vi "Construct.vi"(6 "1553 channel handles":T1[](array[typedef]) {"messages"."timestamps" format="%.0x"; "messages"."parameters"."RxBC channel handle" format="%.0x"; "messages"."parameters"."RxRT channel handle" format="%.0x"; "messages"."parameters"."Tx channel handle" format="%.0x"}, 8 "error in":errorcluster, 9 "1553 channels":T5[](array[typedef]), 10 "id":string, 11 "Execution Unit Implementation":refnum<class "Execution Unit.lvclass">) -> (0 "error out":errorcluster, 3 "Execution Unit Implementation out":refnum<class "Execution Unit.lvclass">)   [LabVIEW 2020, in "Ballard MIL-STD-1553 Engine.lvlib" / "Implementation.lvlib" / "Execution Unit.lvclass"]
uses:
  Execution Unit.lvclass
  Shared/1553 Channel.ctl
  Shared/Terminal Name and Address.ctl
  Shared/Address.ctl
  Shared/Message Definition.ctl
  Shared/Message Type.ctl
  Shared/Terminal Endpoint.ctl
  Shared/Parameter Definition.ctl
  Execution Unit.lvclass/Execution Unit.ctl
  <vilib>/NI VeriStand/Custom Device API/Custom Device Item Ref.ctl
  <vilib>/NI VeriStand/Custom Device API/Custom Device API.lvlib
  Parameter Handles.ctl
  Message Handles.ctl
  1553 Channel Handles.ctl
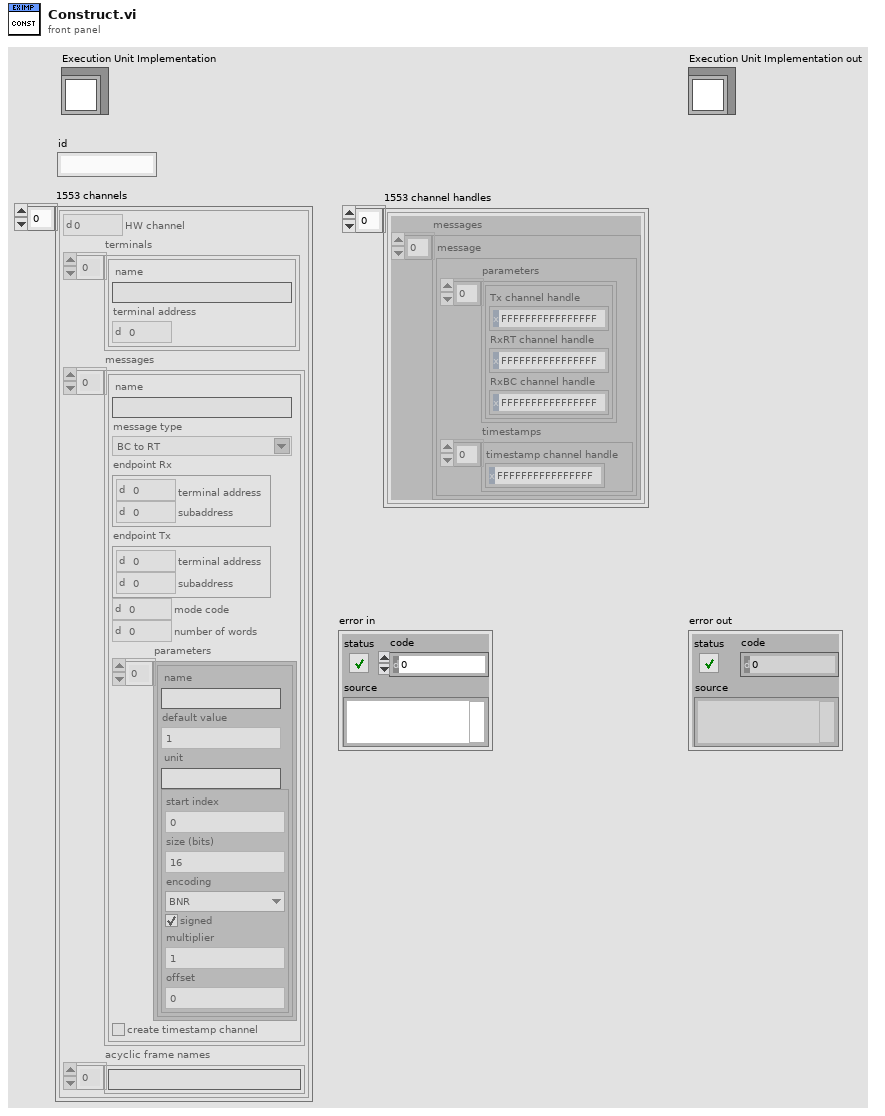
[diagram p1: front panel]
types:
  T1 = typedef "Ballard MIL-STD-1553 Engine.lvlib/Implementation.lvlib/Execution Unit.lvclass/1553 Channel Handles.ctl" = cluster{"messages":T2[]}
  T2 = typedef "Ballard MIL-STD-1553 Engine.lvlib/Implementation.lvlib/Execution Unit.lvclass/Message Handles.ctl" = cluster{"parameters":T3[], "timestamps":T4[]}
  T3 = typedef "Ballard MIL-STD-1553 Engine.lvlib/Implementation.lvlib/Execution Unit.lvclass/Parameter Handles.ctl" = cluster{"Tx channel handle":T4, "RxRT channel handle":T4, "RxBC channel handle":T4}
  T4 = typedef "Custom Device API.lvlib/Custom Device Item Ref.ctl" = u64
  T5 = typedef "1553 Channel.ctl" = cluster{"HW channel":u16, "terminals":T6[], "messages":T8[], "acyclic frame names":string[]}
  T6 = typedef "Terminal Name and Address.ctl" = cluster{"name":string, "terminal address":T7}
  T7 = typedef "Address.ctl" = u16
  T8 = typedef "Message Definition.ctl" = cluster{"name":string, "message type":T9, "endpoint Rx":T10, "endpoint Tx":T10, "mode code":u16, "number of words":u16, "parameters":cluster{"name":string, "default value":dbl, "unit":string, "parameter definition":T11}[], "create timestamp channel":bool}
  T9 = typedef "Message Type.ctl" = string
  T10 = typedef "Terminal Endpoint.ctl" = cluster{"terminal address":T7, "subaddress":T7}
  T11 = typedef "Parameter Definition.ctl" = cluster{"start index":i32, "size (bits)":i32, "encoding":enum16{"BNR", "BCD", "Discrete"}, "signed":bool, "multiplier":dbl, "offset":dbl}
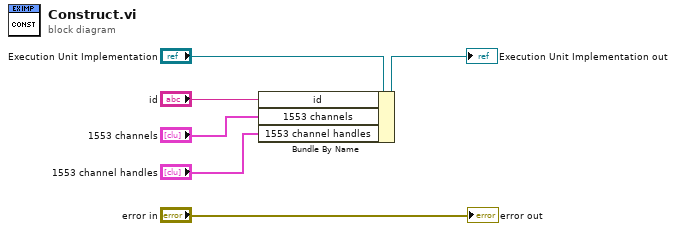
[diagram p0: block diagram]
diagram:
  n1 = Bundle By Name(cluster="Execution Unit Implementation", "id"="id", "1553 channels"="1553 channels", "1553 channel handles"="1553 channel handles") -> (→"Execution Unit Implementation out":refnum<class "Execution Unit.lvclass">)
  "error out" <- "error in"
